vi "Configuration (Read).vi"   [LabVIEW 2013, in "Mercury iXX.lvlib"]
doc: "Read configuration data of the Mercury instrument or any devices within the system."
uses:
  <instrlib>/Mercury iXX/Mercury iXX.lvlib
  <instrlib>/Mercury iXX/Public/Libraries/System.lvlib
  <instrlib>/Mercury iXX/Public/Libraries/Temperature.lvlib
  <instrlib>/Mercury iXX/Public/Libraries/Heater.lvlib
  <instrlib>/Mercury iXX/Public/Libraries/Level Meter.lvlib
  <instrlib>/Mercury iXX/Public/Libraries/Control Loop.lvlib
  <instrlib>/Mercury iXX/Public/Libraries/Auxiliary.lvlib
  <instrlib>/Mercury iXX/Public/Libraries/Magnet.lvlib
  <instrlib>/Mercury iXX/Public/Libraries/Flow.lvlib
  <instrlib>/Mercury iXX/Public/Libraries/Pressure.lvlib
  <instrlib>/Mercury iXX/Public/Libraries/Lambda.lvlib
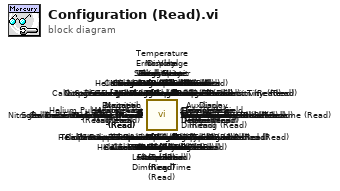
[diagram p0: block diagram]
diagram:
  n1 = call <instrlib>:"Lambda Percentage Flow (Read).vi"() -> ()  [unwired: 7 in, 5 out]
  n2 = call <instrlib>:"Lambda Flow Auto (Read).vi"() -> ()  [unwired: 8 in, 4 out]
  n3 = call <instrlib>:"Helium Pulse Slow-Fast (Read).vi"() -> ()  [unwired: 8 in, 4 out]
  n4 = call <instrlib>:"Temperature Limit (Read).vi"() -> ()  [unwired: 7 in, 5 out]
  n5 = call <instrlib>:"Level Limit (Read).vi"() -> ()  [unwired: 7 in, 5 out]
  n6 = call <instrlib>:"Display Brightness (Read).vi"() -> ()  [unwired: 8 in, 4 out]
  n7 = call <instrlib>:"Display Automatic Dimming Time (Read).vi"() -> ()  [unwired: 8 in, 4 out]
  n8 = call <instrlib>:"Display Automatic Dimming (Read).vi"() -> ()  [unwired: 8 in, 4 out]
  n9 = call <instrlib>:"Nickname (Read).vi"() -> ()  [unwired: 8 in, 4 out]
  n10 = call <instrlib>:"Nickname (Read).vi"() -> ()  [unwired: 8 in, 4 out]
  n11 = call <instrlib>:"PSU Action Status (Read).vi"() -> ()  [unwired: 8 in, 4 out]
  n12 = call <instrlib>:"Serial Number (Read).vi"() -> ()  [unwired: 8 in, 4 out]
  n13 = call <instrlib>:"Pressure Sensor (Read).vi"() -> ()  [unwired: 8 in, 4 out]
  n14 = call <instrlib>:"Pressure Device (Read).vi"() -> ()  [unwired: 8 in, 4 out]
  n15 = call <instrlib>:"Nickname (Read).vi"() -> ()  [unwired: 8 in, 4 out]
  n16 = call <instrlib>:"HVer (Read).vi"() -> ()  [unwired: 8 in, 4 out]
  n17 = call <instrlib>:"FVer (Read).vi"() -> ()  [unwired: 8 in, 4 out]
  n18 = call <instrlib>:"Calibration Scaling (Read).vi"() -> ()  [unwired: 7 in, 5 out]
  n19 = call <instrlib>:"Calibration Offset (Read).vi"() -> ()  [unwired: 8 in, 4 out]
  n20 = call <instrlib>:"Calibration Low Limit (Read).vi"() -> ()  [unwired: 7 in, 5 out]
  n21 = call <instrlib>:"Calibration LastCal (Read).vi"() -> ()  [unwired: 8 in, 4 out]
  n22 = call <instrlib>:"Calibration Interpolation (Read).vi"() -> ()  [unwired: 8 in, 4 out]
  n23 = call <instrlib>:"Calibration High Limit (Read).vi"() -> ()  [unwired: 7 in, 5 out]
  n24 = call <instrlib>:"Calibration Filename (Read).vi"() -> ()  [unwired: 8 in, 4 out]
  n25 = call <instrlib>:"Voltage Limit (Read).vi"() -> ()  [unwired: 7 in, 5 out]
  n26 = call <instrlib>:"Serial Number (Read).vi"() -> ()  [unwired: 8 in, 4 out]
  n27 = call <instrlib>:"Nominal Resistance (Read).vi"() -> ()  [unwired: 7 in, 5 out]
  n28 = call <instrlib>:"Nickname (Read).vi"() -> ()  [unwired: 8 in, 4 out]
  n29 = call <instrlib>:"Maximum Power (Read).vi"() -> ()  [unwired: 7 in, 5 out]
  n30 = call <instrlib>:"HVer (Read).vi"() -> ()  [unwired: 8 in, 4 out]
  n31 = call <instrlib>:"FVer (Read).vi"() -> ()  [unwired: 8 in, 4 out]
  n32 = call <instrlib>:"Flow Device (Read).vi"() -> ()  [unwired: 8 in, 4 out]
  n33 = call <instrlib>:"Fastcool Mode (Read).vi"() -> ()  [unwired: 8 in, 4 out]
  n34 = call <instrlib>:"Calibrate (Read).vi"() -> ()  [unwired: 8 in, 4 out]
  n35 = call <instrlib>:"Calibration LastCal (Read).vi"() -> ()  [unwired: 8 in, 4 out]
  n36 = call <instrlib>:"Flow Auto (Read).vi"() -> ()  [unwired: 8 in, 4 out]
  n37 = call <instrlib>:"Percentage Flow (Read).vi"() -> ()  [unwired: 7 in, 5 out]
  n38 = call <instrlib>:"Sweep Mode (Read).vi"() -> ()  [unwired: 8 in, 4 out]
  n39 = call <instrlib>:"Sweep Table Filename (Read).vi"() -> ()  [unwired: 8 in, 4 out]
  n40 = call <instrlib>:"Target Heater Table Filename (Read).vi"() -> ()  [unwired: 8 in, 4 out]
  n41 = call <instrlib>:"Auto PID Filename (Read).vi"() -> ()  [unwired: 8 in, 4 out]
  n42 = call <instrlib>:"Ignore Voltage Transient Time (Read).vi"() -> ()  [unwired: 7 in, 5 out]
  n43 = call <instrlib>:"Software Voltage Limit (Read).vi"() -> ()  [unwired: 7 in, 5 out]
  n44 = call <instrlib>:"Switch Heater Current (Read).vi"() -> ()  [unwired: 7 in, 5 out]
  n45 = call <instrlib>:"Switch Present (Read).vi"() -> ()  [unwired: 8 in, 4 out]
  n46 = call <instrlib>:"Magnetic Inductance (Read).vi"() -> ()  [unwired: 7 in, 5 out]
  n47 = call <instrlib>:"Current to Field Factor (Read).vi"() -> ()  [unwired: 7 in, 5 out]
  n48 = call <instrlib>:"Current Limit (Read).vi"() -> ()  [unwired: 7 in, 5 out]
  n49 = call <instrlib>:"Output Configuration (Read).vi"() -> ()  [unwired: 8 in, 4 out]
  n50 = call <instrlib>:"Magnet Device (Read).vi"() -> ()  [unwired: 8 in, 4 out]
  n51 = call <instrlib>:"Bipolar Output (Read).vi"() -> ()  [unwired: 8 in, 4 out]
  n52 = call <instrlib>:"Nickname (Read).vi"() -> ()  [unwired: 8 in, 4 out]
  n53 = call <instrlib>:"Serial Number (Read).vi"() -> ()  [unwired: 8 in, 4 out]
  n54 = call <instrlib>:"FVer (Read).vi"() -> ()  [unwired: 8 in, 4 out]
  n55 = call <instrlib>:"HVer (Read).vi"() -> ()  [unwired: 8 in, 4 out]
  n56 = call <instrlib>:"Stepper Speed (Read).vi"() -> ()  [unwired: 7 in, 5 out]
  n57 = call <instrlib>:"Valve Gearing (Read).vi"() -> ()  [unwired: 7 in, 5 out]
  n58 = call <instrlib>:"Temperature Error Voltage Sensitivity (Read).vi"() -> ()  [unwired: 7 in, 5 out]
  n59 = call <instrlib>:"Temperature Error Sensitivity (Read).vi"() -> ()  [unwired: 7 in, 5 out]
  n60 = call <instrlib>:"Gas Flow Scaling (Read).vi"() -> ()  [unwired: 7 in, 5 out]
  n61 = call <instrlib>:"Minimum Gas Flow (Read).vi"() -> ()  [unwired: 7 in, 5 out]
  n62 = call <instrlib>:"Serial Number (Read).vi"() -> ()  [unwired: 8 in, 4 out]
  n63 = call <instrlib>:"FVer (Read).vi"() -> ()  [unwired: 8 in, 4 out]
  n64 = call <instrlib>:"HVer (Read).vi"() -> ()  [unwired: 8 in, 4 out]
  n65 = call <instrlib>:"Aux Device (Read).vi"() -> ()  [unwired: 8 in, 4 out]
  n66 = call <instrlib>:"D Value (Read).vi"() -> ()  [unwired: 7 in, 5 out]
  n67 = call <instrlib>:"I Value (Read).vi"() -> ()  [unwired: 7 in, 5 out]
  n68 = call <instrlib>:"P Value (Read).vi"() -> ()  [unwired: 7 in, 5 out]
  n69 = call <instrlib>:"PID (Read).vi"() -> ()  [unwired: 8 in, 4 out]
  n70 = call <instrlib>:"PID Auto (Read).vi"() -> ()  [unwired: 8 in, 4 out]
  n71 = call <instrlib>:"Temperature Setpoint (Read).vi"() -> ()  [unwired: 7 in, 5 out]
  n72 = call <instrlib>:"Percentage Heat (Read).vi"() -> ()  [unwired: 7 in, 5 out]
  n73 = call <instrlib>:"Heater Auto (Read).vi"() -> ()  [unwired: 8 in, 4 out]
  n74 = call <instrlib>:"Level Association (Read).vi"() -> ()  [unwired: 8 in, 4 out]
  n75 = call <instrlib>:"Auxiliary Association (Read).vi"() -> ()  [unwired: 8 in, 4 out]
  n76 = call <instrlib>:"Heater Association (Read).vi"() -> ()  [unwired: 8 in, 4 out]
  n77 = call <instrlib>:"Control Loop (Read).vi"() -> ()  [unwired: 8 in, 4 out]
  n78 = call <instrlib>:"Nitrogen Pulse Count Period (Read).vi"() -> ()  [unwired: 7 in, 5 out]
  n79 = call <instrlib>:"Helium Probe Resistance (Read).vi"() -> ()  [unwired: 7 in, 5 out]
  n80 = call <instrlib>:"Nitrogen Probe Frequency (Read).vi"() -> ()  [unwired: 7 in, 5 out]
  n81 = call <instrlib>:"Nitrogen Freq at 100 (Read).vi"() -> ()  [unwired: 7 in, 5 out]
  n82 = call <instrlib>:"Nitrogen Freq at 0 (Read).vi"() -> ()  [unwired: 7 in, 5 out]
  n83 = call <instrlib>:"Helium Pulse Delay (Read).vi"() -> ()  [unwired: 7 in, 5 out]
  n84 = call <instrlib>:"Helium Pulse Duration (Read).vi"() -> ()  [unwired: 7 in, 5 out]
  n85 = call <instrlib>:"Helium Pulse Mag (Read).vi"() -> ()  [unwired: 7 in, 5 out]
  n86 = call <instrlib>:"Helium Pre Pulse Duration (Read).vi"() -> ()  [unwired: 7 in, 5 out]
  n87 = call <instrlib>:"Helium Pre Pulse Mag (Read).vi"() -> ()  [unwired: 7 in, 5 out]
  n88 = call <instrlib>:"Helium Resistance at 100 (Read).vi"() -> ()  [unwired: 7 in, 5 out]
  n89 = call <instrlib>:"Helium Resistance at 0 (Read).vi"() -> ()  [unwired: 7 in, 5 out]
  n90 = call <instrlib>:"Serial Number (Read).vi"() -> ()  [unwired: 8 in, 4 out]
  n91 = call <instrlib>:"FVer (Read).vi"() -> ()  [unwired: 8 in, 4 out]
  n92 = call <instrlib>:"HVer (Read).vi"() -> ()  [unwired: 8 in, 4 out]
  n93 = call <instrlib>:"Level Meter Device (Read).vi"() -> ()  [unwired: 8 in, 4 out]
  n94 = call <instrlib>:"Mode (Read).vi"() -> ()  [unwired: 8 in, 4 out]
  n95 = call <instrlib>:"FVer (Read).vi"() -> ()  [unwired: 8 in, 4 out]
  n96 = call <instrlib>:"HVer (Read).vi"() -> ()  [unwired: 8 in, 4 out]
  n97 = call <instrlib>:"Serial Number (Read).vi"() -> ()  [unwired: 8 in, 4 out]
  n98 = call <instrlib>:"HVer (Read).vi"() -> ()  [unwired: 8 in, 4 out]
  n99 = call <instrlib>:"FVer (Read).vi"() -> ()  [unwired: 8 in, 4 out]
  n100 = call <instrlib>:"Maximum Power (Read).vi"() -> ()  [unwired: 7 in, 5 out]
  n101 = call <instrlib>:"Nominal Resistance (Read).vi"() -> ()  [unwired: 7 in, 5 out]
  n102 = call <instrlib>:"Voltage Limit (Read).vi"() -> ()  [unwired: 7 in, 5 out]
  n103 = call <instrlib>:"Nickname (Read).vi"() -> ()  [unwired: 8 in, 4 out]
  n104 = call <instrlib>:"Serial Number (Read).vi"() -> ()  [unwired: 8 in, 4 out]
  n105 = call <instrlib>:"FVer (Read).vi"() -> ()  [unwired: 8 in, 4 out]
  n106 = call <instrlib>:"HVer (Read).vi"() -> ()  [unwired: 8 in, 4 out]
  n107 = call <instrlib>:"Heater Device (Read).vi"() -> ()  [unwired: 8 in, 4 out]
  n108 = call <instrlib>:"Temperature Device (Read).vi"() -> ()  [unwired: 8 in, 4 out]
  n109 = call <instrlib>:"Calibration Cold Limit (Read).vi"() -> ()  [unwired: 7 in, 5 out]
  n110 = call <instrlib>:"Calibration Hot Limit (Read).vi"() -> ()  [unwired: 7 in, 5 out]
  n111 = call <instrlib>:"Calibration Offset (Read).vi"() -> ()  [unwired: 8 in, 4 out]
  n112 = call <instrlib>:"Calibration Scaling (Read).vi"() -> ()  [unwired: 7 in, 5 out]
  n113 = call <instrlib>:"Calibration Interpolation (Read).vi"() -> ()  [unwired: 8 in, 4 out]
  n114 = call <instrlib>:"Calibration Filename (Read).vi"() -> ()  [unwired: 8 in, 4 out]
  n115 = call <instrlib>:"Excitation Magnitude (Read).vi"() -> ()  [unwired: 7 in, 5 out]
  n116 = call <instrlib>:"Excitation Type (Read).vi"() -> ()  [unwired: 8 in, 4 out]
  n117 = call <instrlib>:"Temperature Sensor (Read).vi"() -> ()  [unwired: 8 in, 4 out]
  n118 = call <instrlib>:"Nickname (Read).vi"() -> ()  [unwired: 8 in, 4 out]
  n119 = call <instrlib>:"Serial Number (Read).vi"() -> ()  [unwired: 8 in, 4 out]
  n120 = call <instrlib>:"Time (Read).vi"() -> ()  [unwired: 8 in, 4 out]
  n121 = call <instrlib>:"Flash Space (Read).vi"() -> ()  [unwired: 8 in, 4 out]
  n122 = call <instrlib>:"DateTime (Read).vi"() -> ()  [unwired: 8 in, 4 out]
  n123 = call <instrlib>:"Date (Read).vi"() -> ()  [unwired: 8 in, 4 out]
  n124 = call <instrlib>:"Catalogue (Read).vi"() -> ()  [unwired: 8 in, 4 out]
